vi "Get Queues.vi"(11 "Queues in":refnum<class "Queues.lvclass">) -> (2 "Queues":T1)   [LabVIEW 2021, in "jettl.lvlib" / "jettl Queue Actor.lvlib" / "Queues.lvclass"]
uses:
  Queues.lvclass
  Queues.ctl
  Actor/Msg/Msg.lvclass
  Queues.lvclass/Queues.ctl
  jettl Queue Actor.lvlib
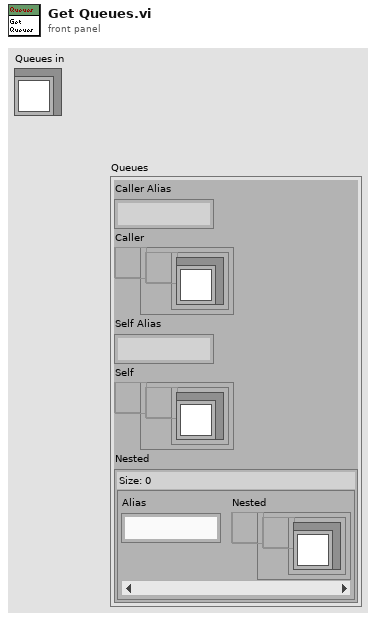
[diagram p1: front panel]
types:
  T1 = typedef "jettl.lvlib/jettl Queue Actor.lvlib/Queues.ctl" = cluster{"Caller Alias":string, "Caller":refnum<data-value>, "Self Alias":string, "Self":refnum<data-value>, "Nested":map{string, refnum<data-value>}}
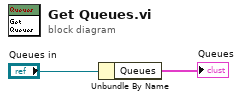
[diagram p0: block diagram]
diagram:
  n1 = Unbundle By Name("Queues in") -> ("Queues"=→"Queues":T1)
